vi "V1_moveby_commands.vi"(6 "case selector":i16[](array[numeric]), 8 "error in (no error)":errorcluster, 9 "even channels":i32[](array[numeric]), 10 "odd channels":i32[](array[numeric]), 11 ".NET Refnum in":refnum<k24>) -> (0 "error out":errorcluster, 3 ".NET Refnum out":refnum<k24>)   [LabVIEW 2020]
uses:
  C:/Users/359167/Documents/LabVIEW_ws/Thorlabs.MotionControl.KCube.InertialMotorCLI.dll
  Thorlabs.MotionControl.KCube.InertialMotorCLI.dll
panel:
  out "# of mounts":dbl
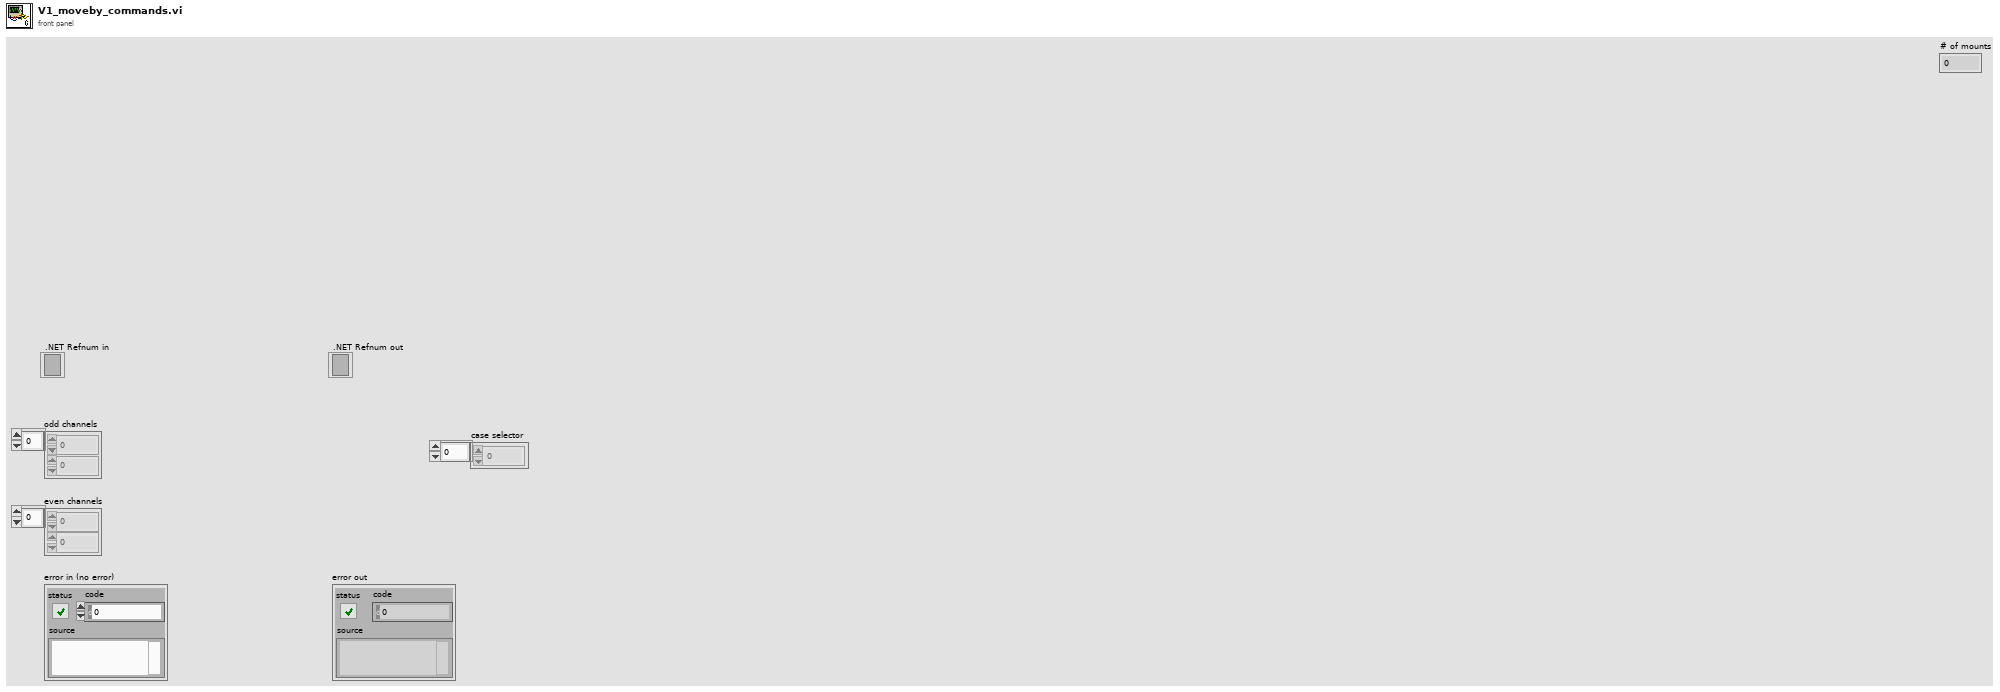
[diagram p1: front panel]
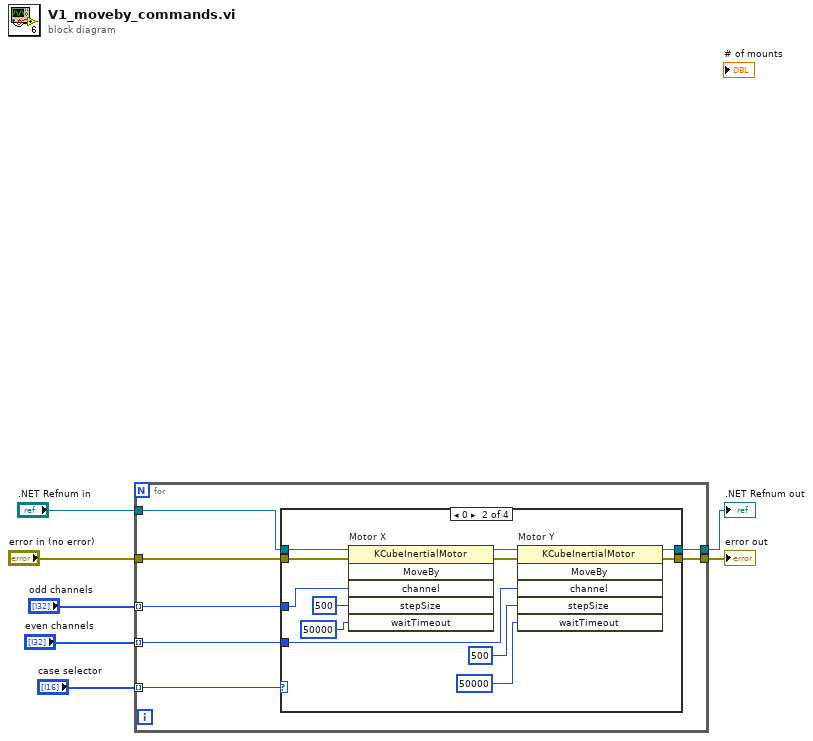
[diagram p0: block diagram]
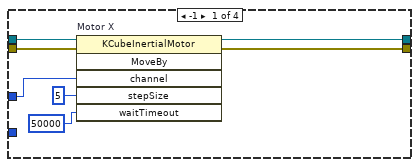
[diagram p2: hidden frame]
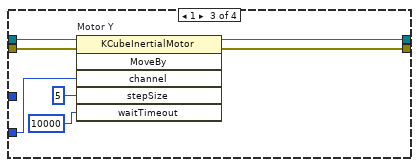
[diagram p3: hidden frame]
diagram:
  n1 = for {
    tunnel: ".NET Refnum in" -> [w14]
    tunnel: [w11] -> w6
    tunnel: "error in (no error)" -> [w13]
    tunnel: [w12] -> w7
    tunnel: "odd channels" -> [w10] mode=indexing
    tunnel: "even channels" -> [w9] mode=indexing
    tunnel: "case selector" -> [w8] mode=indexing
    n2 = case shown="0" w8 {
      tunnel: w14 -> [w17 w33 w38 w41]
      tunnel: [w19 w28 w36 w41] -> w11
      tunnel: [w20 w27 w37 w42] -> w12
      tunnel: w13 -> [w18 w32 w39 w42]
      tunnel: w10 -> [w16 w30 _ _]
      tunnel: w9 -> [_ w25 w35 _]
      frame -1 {
        n3 = invoke on="Motor X" class="KCubeInertialMotor" method="MoveBy"(reference=w17, error in=w18, "channel"=w16, "stepSize"=5, "waitTimeout"=50000) -> (reference out=w19:refnum<k24>, error out=w20:errorcluster)  [unwired: 1 in, 4 out]
      }
      frame 0 {
        n4 = invoke on="Motor X" class="KCubeInertialMotor" method="MoveBy"(reference=w33, error in=w32, "channel"=w30, "stepSize"=500, "waitTimeout"=50000) -> (reference out=w29:refnum<k24>, error out=w26:errorcluster)  [unwired: 1 in, 4 out]
        n5 = invoke on="Motor Y" class="KCubeInertialMotor" method="MoveBy"(reference=w29, error in=w26, "channel"=w25, "stepSize"=500, "waitTimeout"=50000) -> (reference out=w28:refnum<k24>, error out=w27:errorcluster)  [unwired: 1 in, 4 out]
      }
      frame 1 {
        n6 = invoke on="Motor Y" class="KCubeInertialMotor" method="MoveBy"(reference=w38, error in=w39, "channel"=w35, "stepSize"=5, "waitTimeout"=10000) -> (reference out=w36:refnum<k24>, error out=w37:errorcluster)  [unwired: 1 in, 4 out]
      }
      frame 2, Default {
      }
    }
  }
  "error out" <- w7
  ".NET Refnum out" <- w6
